vi "KlingerV2 ConvUnitSgl.vi"(0 "ParamAct":dbl, 5 "UnitDem":u8(ring) caption="Unités\nDemandées" items=["Pas", "mm", "ps", "Degré (°)"], 7 "UnitAct":u8(ring)=2 caption="Unités\nActuelles" items=["Pas", "mm", "ps", "Degré (°)"], 9 "Axe":u8(ring)=3 items=["W", "X", "Y", "Z"], 11 "error in":errorcluster) -> (4 "ParamDem":dbl, 15 "error out":errorcluster)   [LabVIEW 2019]
doc: "Ce VI convertit le nombre spécifié de l'unitée actuelle vers l'unité demandée. Les différentes unité de déplacement disponible sont les pas, les µm et les picosecondes."
uses:
  <userlib>/KlingerV2/KlingerV2 Params.ctl
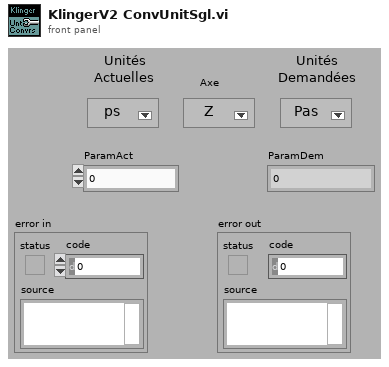
[diagram p1: front panel]
types:
  T1 = typedef "KlingerV2 Params.ctl" = enum16{"Type", "Origine", "Encodeur", "TypeMouv", "FactConv", "Nom", "CorrParams", "KlingCtrlPar", "Speed", "Acc", "Avance", "Tous"}
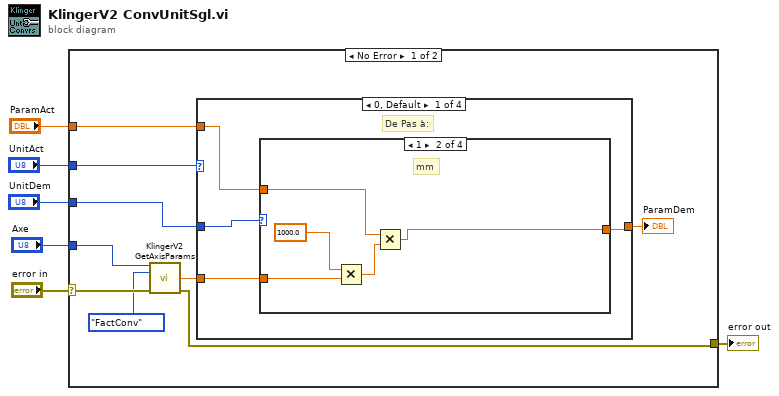
[diagram p0: block diagram]
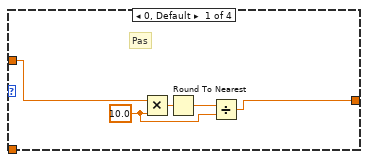
[diagram p2: hidden frame]
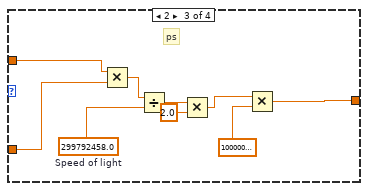
[diagram p3: hidden frame]
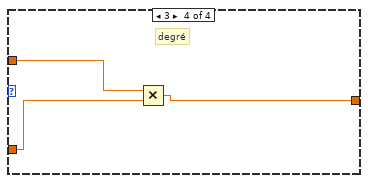
[diagram p4: hidden frame]
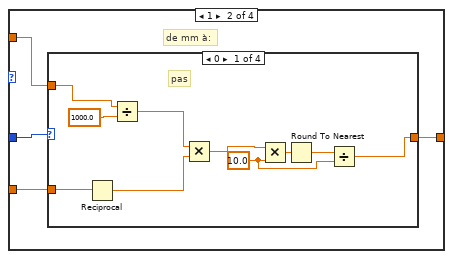
[diagram p5: hidden frame]
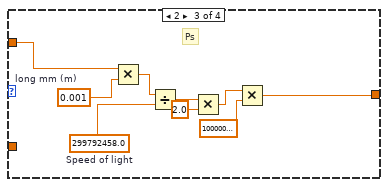
[diagram p7: hidden frame]
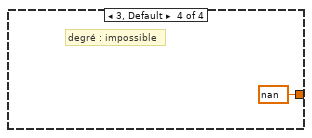
[diagram p8: hidden frame]
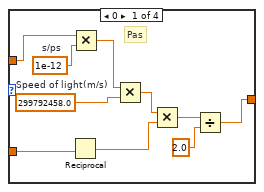
[diagram p10: hidden frame]
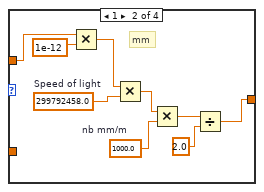
[diagram p11: hidden frame]
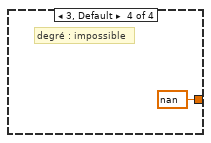
[diagram p12: hidden frame]
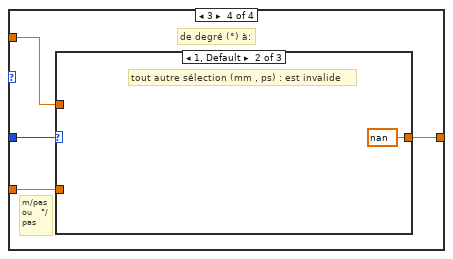
[diagram p13: hidden frame]
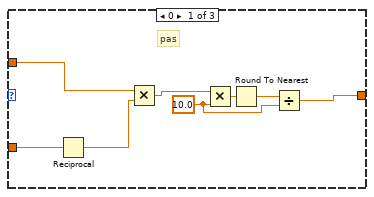
[diagram p14: hidden frame]
diagram:
  n1 = case shown="No Error" "error in" {
    selector: "error in" -> [w13 w106]
    tunnel: [w12 w106] -> w5
    tunnel: "Axe" -> [w10 _]
    tunnel: "ParamAct" -> [w9 _]
    tunnel: "UnitAct" -> [w8 _]
    tunnel: "UnitDem" -> [w7 _]
    frame No Error {
      n2 = call <userlib>:"KlingerV2 GetAxisParams.vi"("Axe"=w10, "Param"=KlingerV2_Params."FactConv", "error in"=w13) -> ("FactConv"=w14:dbl, "error out"=w12:errorcluster)  [unwired: 3 in, 8 out]
      n3 = case shown="0, Default" w8 {
        tunnel: w7 -> [w17 w43 w70 w95]
        tunnel: w9 -> [w18 w45 w69 w94]
        tunnel: [w19 w44 w68 w93] -> w15
        tunnel: w14 -> [w16 w42 w67 w92]
        frame 0, Default {
          # "De Pas à:"
          n4 = case shown="1" w17 {
            tunnel: w18 -> [w21 w29 w34 w41]
            tunnel: [w20 w25 w32 w39] -> w19
            tunnel: w16 -> [_ w26 w30 w40]
            frame 0, Default {
              w22 = 10.0 ("y")
              # "Pas"
              n5 = Multiply(x=w21, y=w22) -> (x*y=w23:dbl)
              n6 = Round To Nearest(number=w23) -> (nearest integer value=w24:dbl)
              n7 = Divide(x=w24, y=w22) -> (x/y=w20:dbl)
            }
            frame 1 {
              # "mm"
              n8 = Multiply(x=1000.0, y=w26) -> (x*y=w27:dbl)
              n9 = Multiply(x=w29, y=w27) -> (x*y=w25:dbl)
            }
            frame 2 {
              w38 = 299792458.0  # Speed of light
              # "ps"
              n10 = Multiply(x=w34, y=w30) -> (x*y=w35:dbl)
              n11 = Divide(x=w35, y=w38) -> (x/y=w37:dbl)
              n12 = Multiply(x=w37, y=2.0) -> (x*y=w33:dbl)
              n13 = Multiply(x=w33, y=1000000000000.0) -> (x*y=w32:dbl)
            }
            frame 3 {
              # "degré"
              n14 = Multiply(x=w41, y=w40) -> (x*y=w39:dbl)
            }
          }
        }
        frame 1 {
          # "de mm à:"
          n15 = case shown="0" w43 {
            tunnel: w45 -> [w53 w56 w60 _]
            tunnel: [w46 w56 w57 nan ("ParamAct")] -> w44
            tunnel: w42 -> [w54 _ _ _]
            frame 0 {
              w48 = 10.0 ("y")
              # "pas"
              n16 = Reciprocal(x=w54) -> (1/x=w55:dbl)
              n17 = Divide(x=w53, y=1000.0) -> (x/y=w51:dbl)
              n18 = Multiply(x=w51, y=w55) -> (x*y=w47:dbl)
              n19 = Multiply(x=w47, y=w48) -> (x*y=w49:dbl)
              n20 = Round To Nearest(number=w49) -> (nearest integer value=w50:dbl)
              n21 = Divide(x=w50, y=w48) -> (x/y=w46:dbl)
            }
            frame 1 {
              # "mm"
            }
            frame 2 {
              w62 = 0.001  # long mm (m)
              w65 = 299792458.0  # Speed of light
              # "Ps"
              n22 = Multiply(x=w60, y=w62) -> (x*y=w61:dbl)
              n23 = Divide(x=w61, y=w65) -> (x/y=w64:dbl)
              n24 = Multiply(x=w64, y=2.0) -> (x*y=w59:dbl)
              n25 = Multiply(x=w59, y=1000000000000.0) -> (x*y=w57:dbl)
            }
            frame 3, Default {
              # "degré : impossible"
            }
          }
        }
        frame 2 {
          # "de Ps à:"
          n26 = case shown="2" w70 {
            tunnel: w69 -> [w74 w82 w90 _]
            tunnel: [w73 w81 w90 nan ("ParamAct")] -> w68
            tunnel: w67 -> [w71 _ _ _]
            frame 0 {
              w76 = 1e-12  # s/ps
              w77 = 299792458.0  # Speed of light(m/s)
              # "Pas"
              n27 = Reciprocal(x=w71) -> (1/x=w72:dbl)
              n28 = Multiply(x=w74, y=w76) -> (x*y=w75:dbl)
              n29 = Multiply(x=w75, y=w77) -> (x*y=w78:dbl)
              n30 = Multiply(x=w78, y=w72) -> (x*y=w80:dbl)
              n31 = Divide(x=w80, y=2.0) -> (x/y=w73:dbl)
            }
            frame 1 {
              w85 = 1000.0  # nb mm/m
              w86 = 299792458.0  # Speed of light
              # "mm"
              n32 = Multiply(x=w82, y=1e-12) -> (x*y=w83:dbl)
              n33 = Multiply(x=w83, y=w86) -> (x*y=w87:dbl)
              n34 = Multiply(x=w87, y=w85) -> (x*y=w89:dbl)
              n35 = Divide(x=w89, y=2.0) -> (x/y=w81:dbl)
            }
            frame 2 {
              # "Ps"
            }
            frame 3, Default {
              # "degré : impossible"
            }
          }
        }
        frame 3 {
          # "m/pas ou   °/pas"
          # "de degré (°) à:"
          n36 = case shown="1, Default" w95 {
            tunnel: w94 -> [w101 _ w105]
            tunnel: [w96 nan ("ParamAct") w105] -> w93
            tunnel: w92 -> [w103 _ _]
            frame 0 {
              w97 = 10.0 ("y")
              # "pas"
              n37 = Reciprocal(x=w103) -> (1/x=w102:dbl)
              n38 = Multiply(x=w101, y=w102) -> (x*y=w98:dbl)
              n39 = Multiply(x=w98, y=w97) -> (x*y=w99:dbl)
              n40 = Round To Nearest(number=w99) -> (nearest integer value=w100:dbl)
              n41 = Divide(x=w100, y=w97) -> (x/y=w96:dbl)
            }
            frame 1, Default {
              # "tout autre sélection (mm , ps) : est invalide"
            }
            frame 3 {
              # "degré"
            }
          }
        }
      }
      "ParamDem" <- w15
    }
    frame Error {
    }
  }
  "error out" <- w5
